vi "Get Info.vi"(8 "error in (no error)":errorcluster, 11 "Report.lvclass in":refnum<class "Wind Report.lvclass">) -> (0 "error out":errorcluster, 1 "Data & Time String":string, 2 "Header":string, 3 "Report.lvclass out":refnum<class "Wind Report.lvclass">, 4 "Data Array":dbl[](array[numeric]), 5 "Pattern":string, 6 "Path":path)   [LabVIEW 2009, in "Wind Report.lvclass"]
doc: "The protected method in the Wind Report class gets the object data for child classes.\n\nAAL 9/09"
uses:
  Wind Report.lvclass
  Wind Report.lvclass/Wind Report.ctl
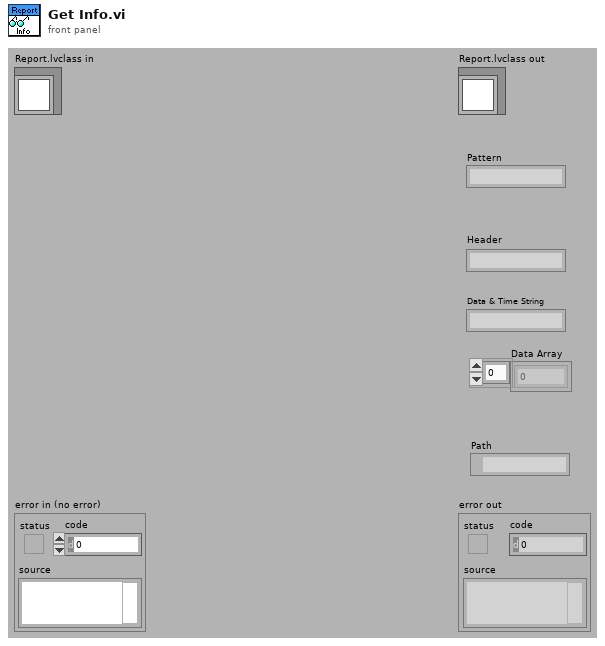
[diagram p1: front panel]
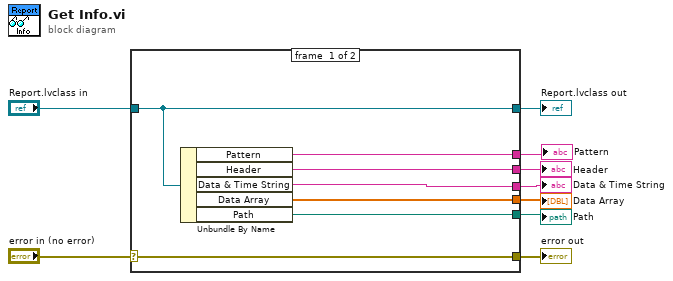
[diagram p0: block diagram]
diagram:
  n1 = case shown="No Error" "error in (no error)" {
    selector: "error in (no error)" -> [w16 w17]
    tunnel: [w16 w17] -> w8
    tunnel: [w15 w18] -> w6
    tunnel: "Report.lvclass in" -> [w15 w18]
    tunnel: [w14 _] -> w5
    tunnel: [w13 _] -> w4
    tunnel: [w12 _] -> w3
    tunnel: [w11 _] -> w2
    tunnel: [w10 _] -> w1
    frame #0 {
      n2 = Unbundle By Name(w15) -> ("Pattern"=w10:string, "Header"=w14:string, "Data & Time String"=w13:string, "Data Array"=w12:dbl[], "Path"=w11:path)
    }
    frame #1 {
    }
  }
  "error out" <- w8
  "Report.lvclass out" <- w6
  "Header" <- w5
  "Data & Time String" <- w4
  "Data Array" <- w3
  "Path" <- w2
  "Pattern" <- w1
